vi "Setj1939.vi"(8 "error in (no error)":errorcluster, 10 "Set_Val":T1, 11 "OneOfTemplate in":refnum<class "nixnet_grpc_FrameBufferResponse_frame.lvclass">) -> (0 "error out":errorcluster, 3 "OneOfTemplate out":refnum<class "nixnet_grpc_FrameBufferResponse_frame.lvclass">)   [LabVIEW 2019, in "xnet-grpc_client.lvlib" / "nixnet_grpc_FrameBufferResponse_frame.lvclass"]
uses:
  nixnet_grpc_FrameBufferResponse_frame.lvclass
  nixnet_grpc_FrameBufferResponse_frame.lvclass/nixnet_grpc_FrameBufferResponse_frame.ctl
  nixnet_grpc_FrameFlags.ctl
  xnet-grpc_client.lvlib
  nixnet_grpc_FrameType.ctl
  nixnet_grpc_FrameResponse.ctl
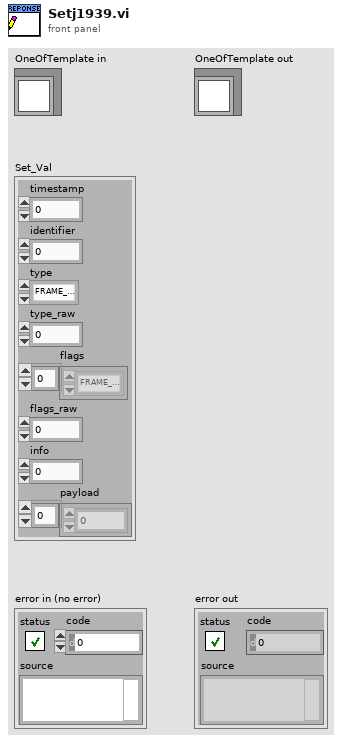
[diagram p1: front panel]
types:
  T1 = typedef "xnet-grpc_client.lvlib/nixnet_grpc_FrameResponse.ctl" = cluster{"timestamp":u64, "identifier":u32, "type":T2, "type_raw":u32, "flags":T3[], "flags_raw":u32, "info":u32, "payload":u8[]}
  T2 = typedef "xnet-grpc_client.lvlib/nixnet_grpc_FrameType.ctl" = enum32{"FRAME_TYPE_CAN_DATA", "FRAME_TYPE_CAN_REMOTE", "FRAME_TYPE_CAN_BUS_ERROR", "FRAME_TYPE_CAN20_DATA", "FRAME_TYPE_CANFD_DATA", "FRAME_TYPE_CANFDBRS_DATA", "FRAME_TYPE_FLEX_RAY_DATA", "FRAME_TYPE_FLEX_RAY_NULL", "FRAME_TYPE_FLEX_RAY_SYMBOL", "FRAME_TYPE_LIN_DATA", "FRAME_TYPE_LIN_BUS_ERROR", "FRAME_TYPE_LIN_NO_RESPONSE", "FRAME_TYPE_J1939_DATA", "FRAME_TYPE_SPECIAL_DELAY", "FRAME_TYPE_SPECIAL_LOG_TRIGGER", "FRAME_TYPE_SPECIAL_START_TRIGGER"}
  T3 = typedef "xnet-grpc_client.lvlib/nixnet_grpc_FrameFlags.ctl" = enum32{"FRAME_FLAGS_UNSPECIFIED", "FRAME_FLAGS_FLEX_RAY_STARTUP", "FRAME_FLAGS_FLEX_RAY_SYNC", "FRAME_FLAGS_FLEX_RAY_PREAMBLE", "FRAME_FLAGS_FLEX_RAY_CH_A", "FRAME_FLAGS_FLEX_RAY_CH_B", "FRAME_FLAGS_LIN_EVENT_SLOT", "FRAME_FLAGS_TRANSMIT_ECHO"}
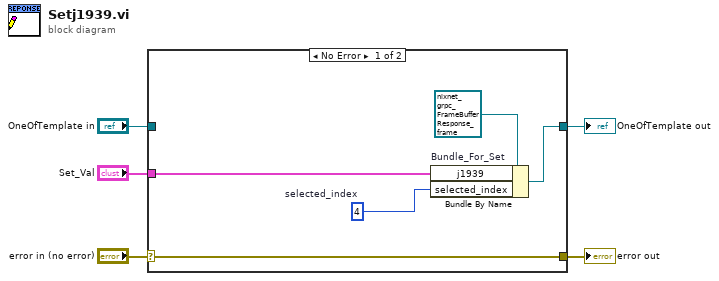
[diagram p0: block diagram]
diagram:
  n1 = case shown="No Error" "error in (no error)" {
    selector: "error in (no error)" -> [w10 w11]
    tunnel: [w10 w11] -> w4
    tunnel: [w9 w12] -> w2
    tunnel: "OneOfTemplate in" -> [_ w12]
    tunnel: "Set_Val" -> [w8 _]
    frame No Error {
      w7 = 4  # selected_index
      n2 = Bundle By Name "Bundle_For_Set"(cluster=refnum<class "nixnet_grpc_FrameBufferResponse_frame.lvclass"> refnum ("OneOfTemplate in"), "j1939"=w8, "selected_index"=w7) -> (w9:refnum<class "nixnet_grpc_FrameBufferResponse_frame.lvclass">)
    }
    frame Error {
    }
  }
  "error out" <- w4
  "OneOfTemplate out" <- w2
